vi "Constructor.vi"(6 "Check Manager":refnum<class "Constraint Manager.lvclass">, 7 "Configuration":refnum<class "Column Configuration.lvclass">, 8 "error in (no error)":errorcluster, 9 "Value Type":refnum<class "Value Type.lvclass">, 10 "Value Source":refnum<class "Value Source.lvclass">, 11 "Composed Column in":refnum<class "Composed Column.lvclass">) -> (0 "error out":errorcluster, 3 "Composed Column out":refnum<class "Composed Column.lvclass">)   [LabVIEW 2020, in "Composed Columns.lvlib" / "Composed Column.lvclass"]
uses:
  Composed Column.lvclass
  Basic Columns/Column Configuration/Basic Column Configuration Class/Column Configuration.lvclass
  Composed Columns/Value Source Interface Class/Value Source.lvclass
  Value Type/Value Type.lvclass
  Check Manager/Constraint Manager.lvclass
  Composed Column.lvclass/Composed Column.ctl
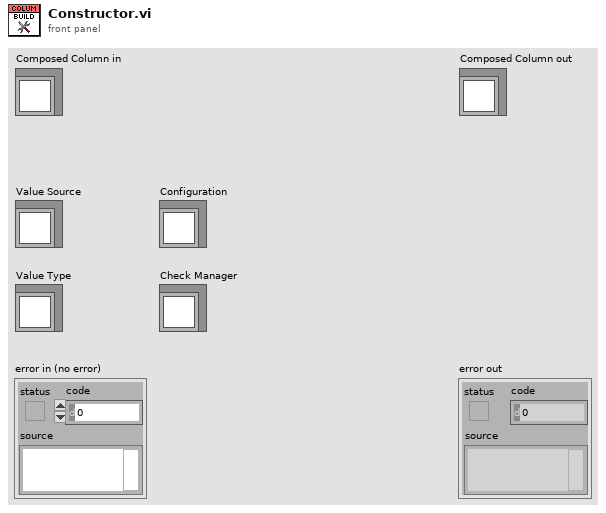
[diagram p1: front panel]
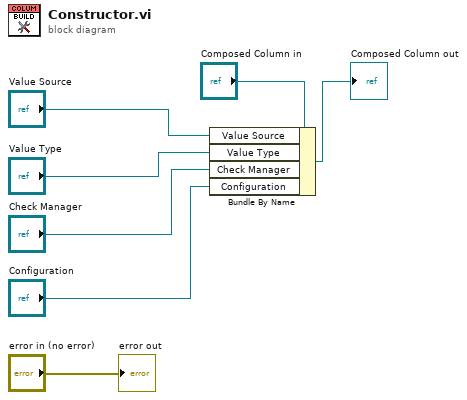
[diagram p0: block diagram]
diagram:
  n1 = Bundle By Name(cluster="Composed Column in", "Value Source"="Value Source", "Value Type"="Value Type", "Check Manager"="Check Manager", "Configuration"="Configuration") -> (→"Composed Column out":refnum<class "Composed Column.lvclass">)
  "error out" <- "error in (no error)"
